vi "Output Snake Coordinates.vi"(11 "Snake in":refnum<class "Snake.lvclass">) -> (2 "Tail":T1[](array[typedef]))   [LabVIEW 2018, in "Snake.lvclass"]
uses:
  Snake.lvclass
  Type Defs/Coordinates.ctl
  Snake.lvclass/Snake.ctl
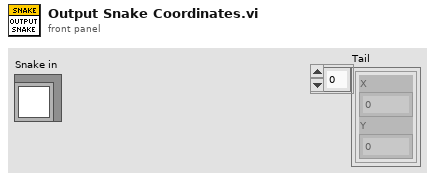
[diagram p1: front panel]
types:
  T1 = typedef "Coordinates.ctl" = cluster{"X":i32, "Y":i32}
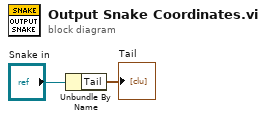
[diagram p0: block diagram]
diagram:
  n1 = Unbundle By Name("Snake in") -> ("Tail"=→"Tail":T1[])
